vi "get_all_crystal_positions.vi"(8 "error in":errorcluster, 10 "7th Crystal?":bool, 11 "address":string) -> (0 "error out":errorcluster, 3 "Crystal Positions Array":i32[](array[numeric]))   [LabVIEW 2020]
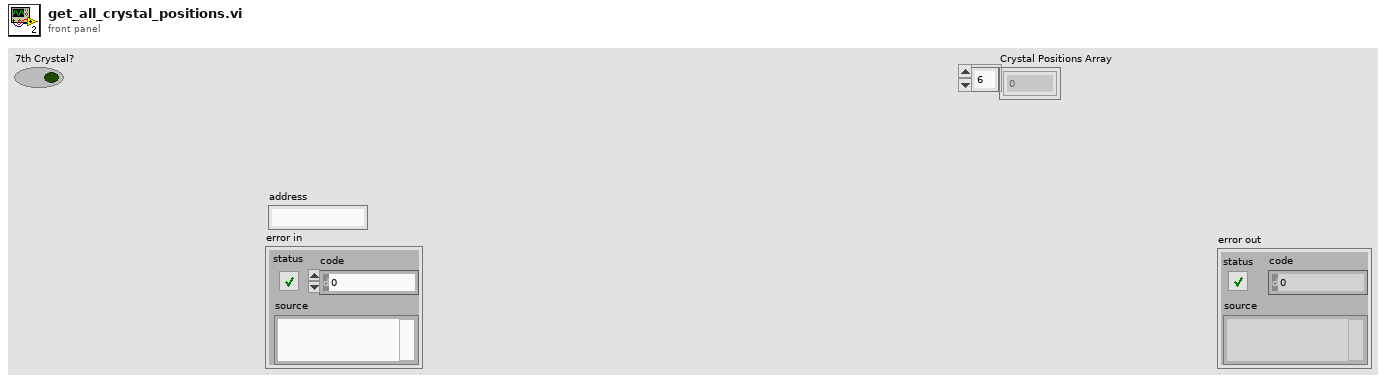
[diagram p1: front panel]
types:
  T1 = enum16{"Standard", "Buffered", "CRLF", "Immediate"}
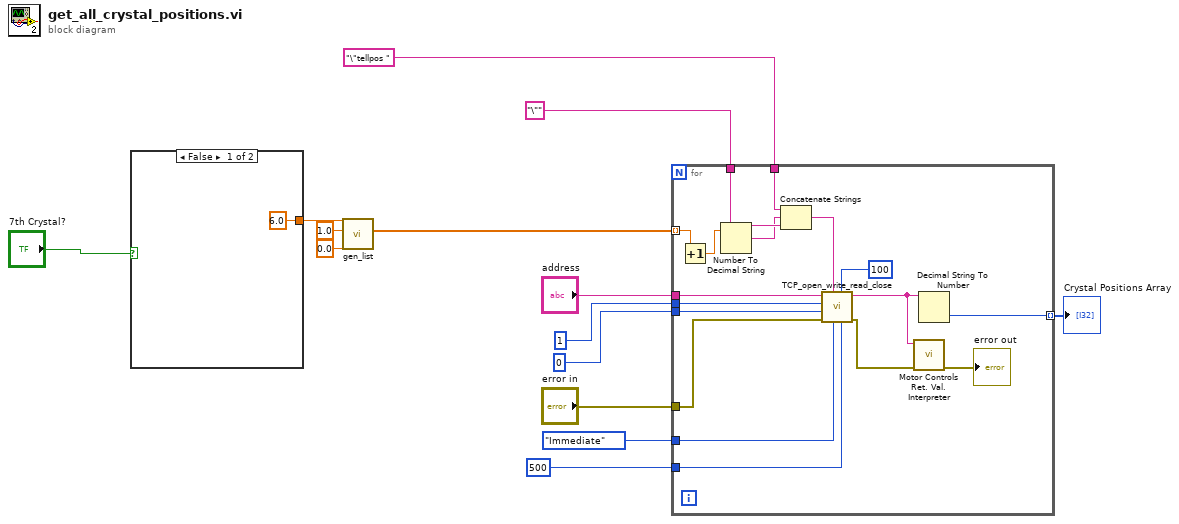
[diagram p0: block diagram]
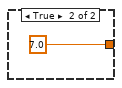
[diagram p2: hidden frame]
diagram:
  n1 = case shown="False" "7th Crystal?" {
    tunnel: [6.0 ("Upper bound") 7.0 ("Upper bound")] -> w5
    frame False {
    }
    frame True {
    }
  }
  n2 = call "gen_list.vi"("Lower Bound"=0.0, "Step Size"=1.0, "Upper bound"=w5) -> ("Array"=w6:dbl[])  [unwired: 8 in]
  n3 = for {
    tunnel: "address" -> [w33]
    tunnel: u16 1 ("remote port or service name") -> [w32]
    tunnel: u16 0 ("local port (0)") -> [w31]
    tunnel: "error in" -> [w30]
    tunnel: T1."Immediate" ("mode (standard)") -> [w29]
    tunnel: 500 ("timeout ms (25000)") -> [w24]
    tunnel: [w23] -> w1 mode=indexing
    tunnel: "\"tellpos " ("write string") -> [w22]
    tunnel: "\"" ("string") -> [w21]
    tunnel: w6 -> [w19] mode=indexing
    n4 = Increment(x=w19) -> (x+1=w18:dbl)
    n5 = Number To Decimal String(number=w18) -> (decimal integer string=w20:string)  [unwired: 1 in]
    n6 = Concatenate Strings(w22, w20, w21) -> (w17:string)
    n7 = call "TCP_open_write_read_close.vi"("timeout ms (25000)"=w24, "bytes to read"=100, "mode (standard)"=w29, "write string"=w17, "error in"=w30, "local port (0)"=w31, "remote port or service name"=w32, "address"=w33) -> ("error out"=w27:errorcluster, "read string"=w25:string)  [unwired: 2 in]
    n8 = call "Motor Controls Ret. Val. Interpreter.vi"("error in"=w27, "Command Return"=w25) -> ("error out"=→"error out":errorcluster)  [unwired: 8 in, 1 out]
    n9 = Decimal String To Number(string=w25) -> (number=w23:i32)  [unwired: 2 in, 1 out]
  }
  "Crystal Positions Array" <- w1
